vi "S2C_PCIe7841_Proc_AnalogReadLocal.vi"(8 "Error In":errorcluster, 9 "ExeRef":refnum<vi>, 11 "Q-Ref":refnum<queue>) -> (0 "Error Out":errorcluster, 3 "Command":string)   [LabVIEW 2015]
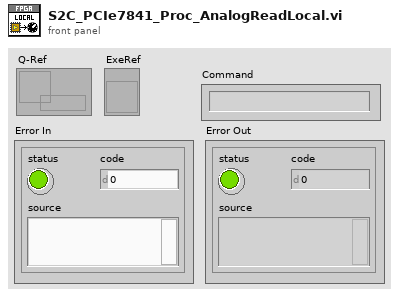
[diagram p1: front panel]
types:
  T1 = cluster{"Caller-Q":refnum<queue>, "Command":string, "Return":string, "Data":variant, "Timeout":dbl}
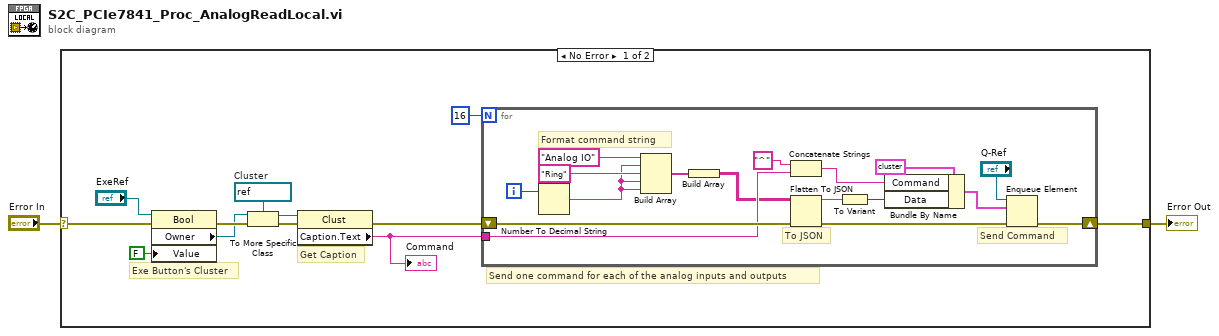
[diagram p0: block diagram]
diagram:
  n1 = case shown="No Error" "Error In" {
    selector: "Error In" -> [w8 w32]
    tunnel: [w6 w32] -> w1
    frame No Error {
      w11 = refnum<vi> refnum  # Cluster
      # "Send one command for each of the analog inputs and outputs"
      # "Get Caption"
      # "Exe Button's Cluster"
      n2 = property class="Bool"(reference="ExeRef", error in=w8, "Value"=FALSE) -> (error out=w13:errorcluster, "Owner"=w12:refnum<vi>)  [unwired: 1 out]
      n3 = To More Specific Class(target class=w11, reference=w12, error in=w13) -> (specific class reference=w9:refnum<vi>, error out=w10:errorcluster)
      n4 = property class="Clust"(reference=w9, error in=w10) -> (error out=w5:errorcluster, "Caption.Text"=w4:string)  [unwired: 1 out]
      "Command" <- w4
      n5 = for {
        N: 16 -> [_]
        shift-right: [w30] -> w6
        shift-left: w5 -> [w31]
        tunnel: w4 -> [w29]
        i -> [w16]
        # "Format command string"
        # "Send Command"
        # "To JSON"
        n6 = Number To Decimal String(number=w16) -> (decimal integer string=w26:string)  [unwired: 1 in]
        n7 = Build Array("Analog IO" ("element"), w26, "Ring", w26, w26) -> (w17:string[])
        n8 = Build Array(w17) -> (w15:string[][])
        n9 = Concatenate Strings("^" ("string"), w29) -> (w21:string)
        n10 = Flatten To JSON(anything=w15, error in (no error)=w31) -> (JSON string=w19:string, 11:w18:errorcluster)  [unwired: 1 in]
        n11 = To Variant(anything=w19) -> (Variant=w23:variant)
        n12 = Bundle By Name(cluster=T1 {"Caller-Q"=refnum, "Command"="", "Return"="None", "Data"=variant, "Timeout"=10.0} ("element"), "Command"=w21, "Data"=w23) -> (w24:T1)
        n13 = Enqueue Element(queue="Q-Ref", element=w24, error in (no error)=w18) -> (error out=w30:errorcluster)  [unwired: 1 in, 2 out]
      }
    }
    frame Error {
    }
  }
  "Error Out" <- w1
